vi "MB Analysis.vi"() -> ()   [LabVIEW 2016]
uses:
  <vilib>/Utility/file.llb/Write Delimited Spreadsheet (string).vi
panel:
  in  "Tab Control 2":enum32{"Calculated Values", "Other Values"}(tab)
  out "System Weight (N)":dbl format="%#_12g"
  out "Peak Force":dbl
  out "Peak Power":dbl
  out "Force at PP":dbl
  out "Velocity at PP":dbl
  out "Peak Velocity":dbl
  out "Peak Acceleration":dbl
  out "Time between R/B Cursors":dbl
  out "System Weight \nCursor Position":dbl
  out "Beginning of\nThrow Cursor\nPosition":dbl
  out "End of Throw\nCursor Position":dbl
  out "Avg Force \nbetween B/R Cursors":dbl
  in  "Tab Control 3":T1(tab)
  out "Measured Segment Force":dbl[](graph)
  out "Measured Segment COM Acceleration":dbl[](graph)
  out "Measured Segment COM Velocity":dbl[](graph)
  out "Measured Segment COM Power":dbl[](graph)
  out "Combined":dbl[][](graph)
  in  "Tab Control":T2(tab)
  in  "Subject Identifier (ID# or Last Name, First)":string
  in  "Medicine Ball Weight":string
  in  "Attempt Number":string
  in  "Save Results":bool
  in  "Create Blank\nEntry File":bool
  in  "Attempt Notes":string
  out "Target File for Saving Results":path
  in  "Choose New \nSave Target":bool
  in  "column in datafile \ncontaining force data":i32=1
  in  "# of Samples Averaged\nfor standing weight\n(1000 is default)":i32=1000 caption="Samples"
  in  "stop":bool
  out "Force-time trace":dynamicdata(graph)
  out "Path":path
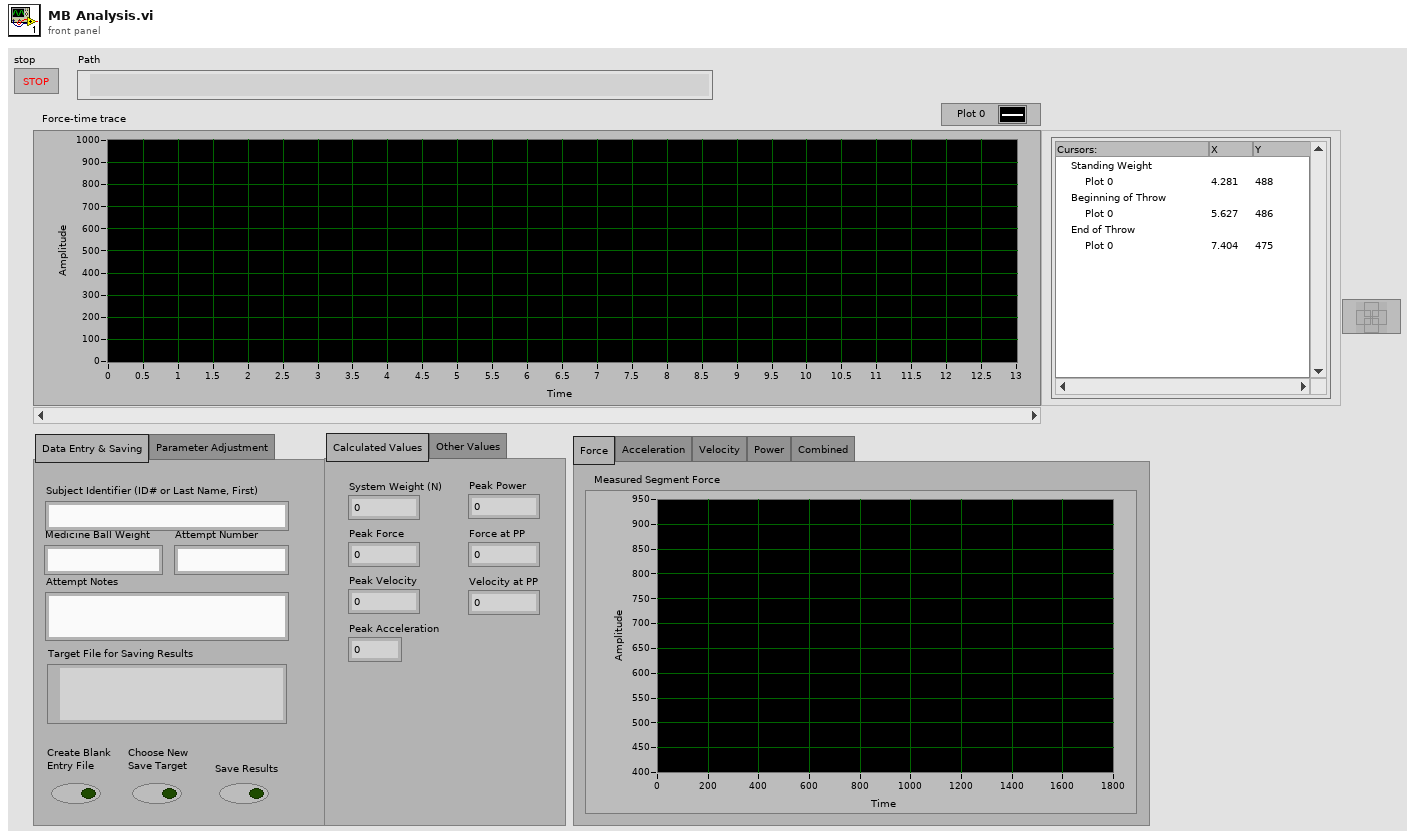
[diagram p1: front panel]
types:
  T1 = enum32{"Force", "Acceleration", "Velocity", "Power", "Combined"}
  T2 = enum32{"Data Entry & Saving", "Parameter Adjustment"}
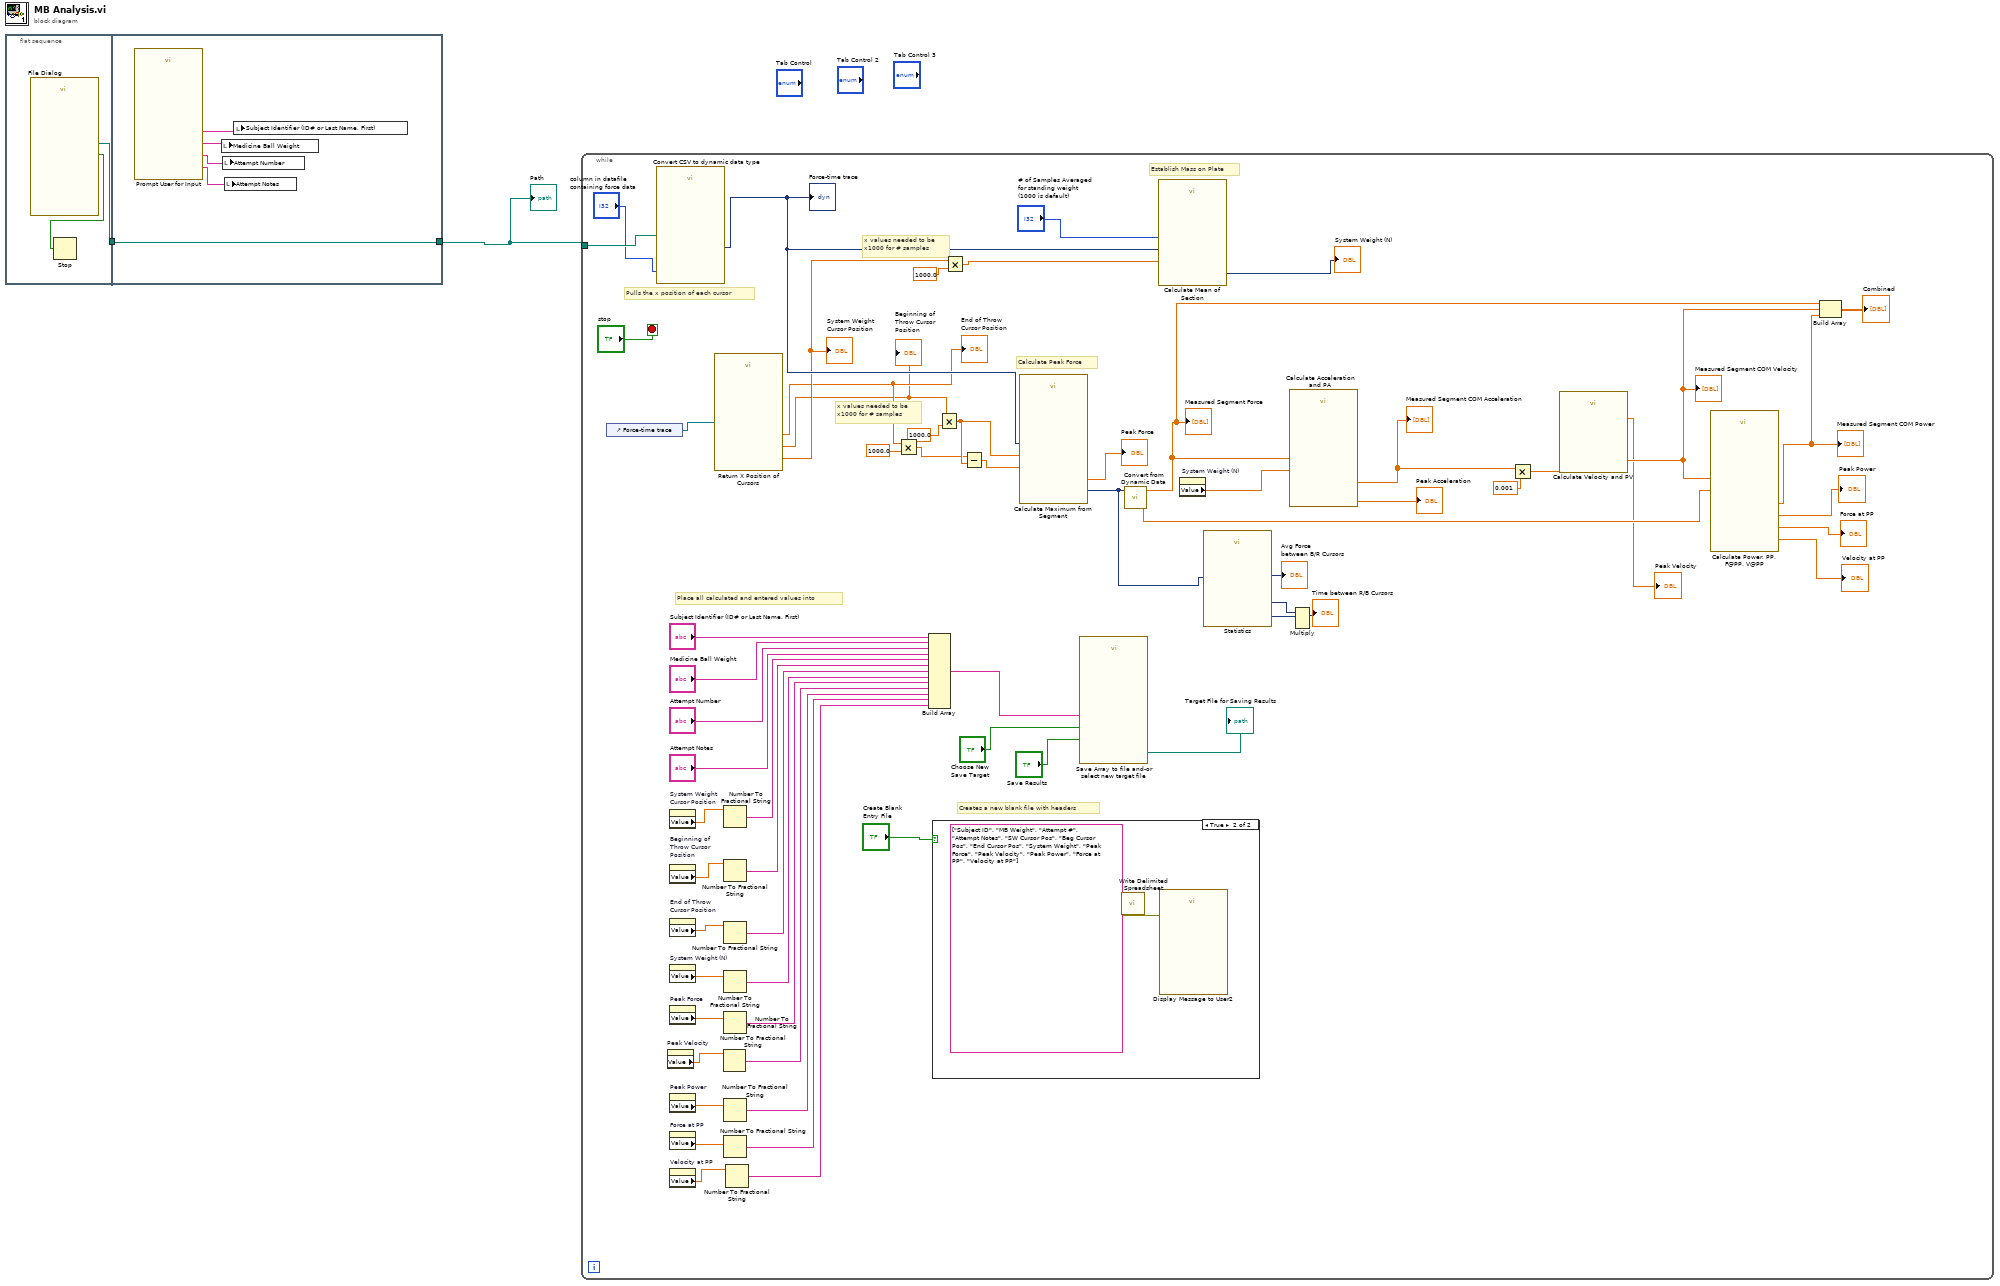
[diagram p0: block diagram]
diagram:
  n1 = flat-sequence {
    tunnel: [w4] -> w2
    tunnel: w2 -> [w5]
    tunnel: [w5] -> w1
    frame #0 {
      n2 = call "File Dialog"() -> ("selected path"=w4:path, "cancelled"=w3:bool)  [unwired: 12 in, 2 out]
      n3 = Stop(stop? (T)=w3) -> ()
    }
    frame #1 {
      n4 = call "Prompt User for Input"() -> ("Attempt Notes"=w8:string, "Attempt Number"=w9:string, "Medicine Ball Weight"=w7:string, "Subject ID or Last Name, First Name"=w6:string)  [unwired: 14 in, 2 out]
      n5 = local write "Medicine Ball Weight"(w7) -> ()
      n6 = local write "Attempt Number"(w9) -> ()
      n7 = local write "Attempt Notes"(w8) -> ()
      n8 = local write "Subject Identifier (ID# or Last Name, First)"(w6) -> ()
    }
  }
  n9 = while {
    tunnel: w1 -> [w71]
    stop <- "stop" stop-if-true
    # "Place all calculated and entered values into"
    # "Creates a new blank file with headers"
    # "x values needed to be \nx1000 for # samples"
    # "x values needed to be \nx1000 for # samples"
    # "Calculate Peak Force"
    # "Establish Mass on Plate"
    # "Pulls the x position of each cursor"
    n10 = control-ref of="Force-time trace"() -> (w70:refnum<vi>)
    n11 = call "Convert CSV to dynamic data type.vi"("column containing\nforce data"="column in datafile \ncontaining force data", "selected path"=w71) -> ("Dynamic Data Type"=w62:dynamicdata)  [unwired: 1 in]
    "Force-time trace" <- w62
    n12 = property on="Peak Velocity" class="DigNum (strict)"() -> ("Value"=w18:dbl)  [unwired: 2 in, 2 out]
    n13 = property on="System Weight \nCursor Position" class="DigNum (strict)"() -> ("Value"=w32:dbl)  [unwired: 2 in, 2 out]
    n14 = property on="Beginning of\nThrow Cursor\nPosition" class="DigNum (strict)"() -> ("Value"=w31:dbl)  [unwired: 2 in, 2 out]
    n15 = property on="End of Throw\nCursor Position" class="DigNum (strict)"() -> ("Value"=w30:dbl)  [unwired: 2 in, 2 out]
    n16 = property on="System Weight (N)" class="DigNum (strict)"() -> ("Value"=w41:dbl)  [unwired: 2 in, 2 out]
    n17 = property on="Peak Force" class="DigNum (strict)"() -> ("Value"=w42:dbl)  [unwired: 2 in, 2 out]
    n18 = property on="Peak Power" class="DigNum (strict)"() -> ("Value"=w40:dbl)  [unwired: 2 in, 2 out]
    n19 = property on="Force at PP" class="DigNum (strict)"() -> ("Value"=w39:dbl)  [unwired: 2 in, 2 out]
    n20 = property on="Velocity at PP" class="DigNum (strict)"() -> ("Value"=w38:dbl)  [unwired: 2 in, 2 out]
    n21 = call "Return X Position of Cursors.vi"("WaveformGraph in"=w70) -> ("Cursor 1 X Pos"=w53:dbl, "Cursor 2 X Pos"=w50:dbl, "Cursor 3 X Pos"=w54:dbl)  [unwired: 8 in]
    "System Weight \nCursor Position" <- w54
    "Beginning of\nThrow Cursor\nPosition" <- w50
    "End of Throw\nCursor Position" <- w53
    n22 = Number To Fractional String(number=w18) -> (F-format string=w19:string)  [unwired: 3 in]
    n23 = Number To Fractional String(number=w32) -> (F-format string=w33:string)  [unwired: 3 in]
    n24 = Number To Fractional String(number=w31) -> (F-format string=w34:string)  [unwired: 3 in]
    n25 = Number To Fractional String(number=w30) -> (F-format string=w35:string)  [unwired: 3 in]
    n26 = Number To Fractional String(number=w41) -> (F-format string=w36:string)  [unwired: 3 in]
    n27 = Number To Fractional String(number=w42) -> (F-format string=w37:string)  [unwired: 3 in]
    n28 = Number To Fractional String(number=w40) -> (F-format string=w20:string)  [unwired: 3 in]
    n29 = Number To Fractional String(number=w39) -> (F-format string=w21:string)  [unwired: 3 in]
    n30 = Number To Fractional String(number=w38) -> (F-format string=w22:string)  [unwired: 3 in]
    n31 = Multiply(x=w53, y=1000.0) -> (x*y=w12:dbl)
    n32 = Build Array("Subject Identifier (ID# or Last Name, First)", "Medicine Ball Weight", "Attempt Number", "Attempt Notes", w33, w34, w35, w36, w37, w19, w20, w21, w22) -> (w45:string[])
    n33 = case shown="True" "Create Blank\nEntry File" {
      frame False {
      }
      frame True {
        # "All labels go here, in order"
        n34 = call-poly <vilib>:"Write Delimited Spreadsheet.vi"("1D data"=string[] ["Subject ID", "MB Weight", "Attempt #", "Attempt Notes", "SW Cursor Pos", "Beg Cursor Pos", "End Cursor Pos", "System Weight", "Peak Force", "Peak Velocity", "Peak Power", "Force at PP", "Velocity at PP"]) -> ("error out"=w73:errorcluster)  [unwired: 13 in, 1 out]
        n35 = call "Display Message to User2"("error in (no error)"=w73) -> ()  [unwired: 9 in, 2 out]
      }
    }
    n36 = Multiply(x=w50, y=1000.0) -> (x*y=w65:dbl)
    n37 = Multiply(x=w54, y=1000.0) -> (x*y=w68:dbl)
    n38 = Subtract(x=w12, y=w65) -> (x-y=w11:dbl)
    n39 = call "Calculate Maximum from Segment.vi"("Sample Number"=w11, "Begin Sample"=w65, "Dynamic Data Type"=w62) -> ("Section"=w10:dynamicdata, "Peak Force"=→"Peak Force":dbl)  [unwired: 7 in]
    n40 = call "Save Array to file and-or select new target file.vi"("Choose New \nSave Target"="Choose New \nSave Target", "Save Results"="Save Results", "Values to Save"=w45) -> ("selected path"=→"Target File for Saving Results":path)  [unwired: 8 in]
    n41 = call "Convert from Dynamic Data"("Dynamic Data Type"=w10) -> ("Array"=w29:dbl[])  [unwired: 3 in]
    "Measured Segment Force" <- w29
    n42 = call "Calculate Mean of Section.vi"("# of Samples Averaged\nfor standing weight\n(500 is default)"="# of Samples Averaged\nfor standing weight\n(1000 is default)", "Start of Sample"=w68, "Dynamic Data Type"=w62) -> ("Average"=→"System Weight (N)":dynamicdata)  [unwired: 8 in]
    n43 = property on="System Weight (N)" class="DigNum (strict)"() -> ("Value"=w63:dbl)  [unwired: 2 in, 2 out]
    n44 = call "Statistics"("Signals"=w10) -> ("Total Samples"=w15:dynamicdata, "Arithmetic Mean"=→"Avg Force \nbetween B/R Cursors":dynamicdata, "Time Delta"=w14:dynamicdata)  [unwired: 23 in, 1 out]
    n45 = call "Calculate Acceleration and PA.vi"("System Weight"=w63, "Force Array"=w29) -> ("Acceleration Array"=w55:dbl[], "Peak Acceleration"=→"Peak Acceleration":dbl)  [unwired: 8 in]
    "Measured Segment COM Acceleration" <- w55
    n46 = Multiply(1:w14, 2:w15) -> (0:→"Time between R/B Cursors":dynamicdata)  [unwired: 1 in, 1 out]
    n47 = Multiply(x=w55, y=0.001) -> (x*y=w61:dbl[])
    n48 = call "Calculate Velocity and PV.vi"("Acceleration Array"=w61) -> ("Peak velocity"=→"Peak Velocity":dbl, "Velocity Array"=w27:dbl[])  [unwired: 9 in]
    "Measured Segment COM Velocity" <- w27
    n49 = call "Calculate Power, PP, F@PP, V@PP.vi"("Velocity Array"=w27, "Force Array"=w29) -> ("Force at PP"=→"Force at PP":dbl, "Peak Power"=→"Peak Power":dbl, "Power Array"=w26:dbl[], "Velocity at PP"=→"Velocity at PP":dbl)  [unwired: 6 in]
    "Measured Segment COM Power" <- w26
    n50 = Build Array(w29, w27, w26) -> (→"Combined":dbl[][])
  }
  "Path" <- w1
